vi "WaveformComponent, Append Pulse Center.vi"(0 "waveform in":waveform(dbl)={"t0"=timestamp(3474820848.0780005 s since 1904-01-01), "dt"=nan, "Y"=[]}, 1 "append parameters":T1={"offset"=0.5, "amplitude"=-2.0, "delay"=0.00019999999999999998, "leading edge"=0.0005, "pulse width"=0.0006, "trailing edge"=0.0005, "ref level %"=33.333} {"ref level %" format="%.3f"; "offset" format="%.3f"; "pulse width" format="%.1f"; "trailing edge" format="%.1f"; "amplitude" format="%.3f"; "delay" format="%.1f"; "leading edge" format="%.1f"}) -> (3 "waveform out":waveform(dbl)={"t0"=timestamp(-9593225999.921999 s since 1904-01-01), "dt"=nan, "Y"=[]})   [LabVIEW 2010]
uses:
  Pulse Parameters.ctl
panel:
  out "edge rate adjustment":dbl[unit] format="%.3p"
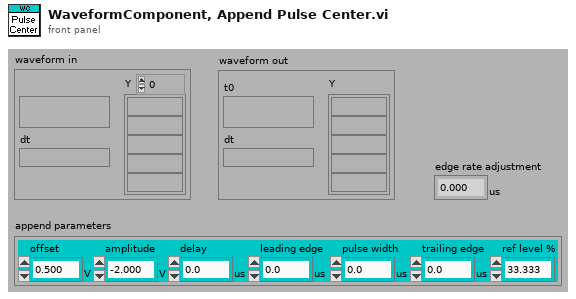
[diagram p1: front panel]
types:
  T1 = typedef "Pulse Parameters.ctl" = cluster{"offset":dbl[unit], "amplitude":dbl[unit], "delay":dbl[unit], "leading edge":dbl[unit], "pulse width":dbl[unit], "trailing edge":dbl[unit], "ref level %":dbl}
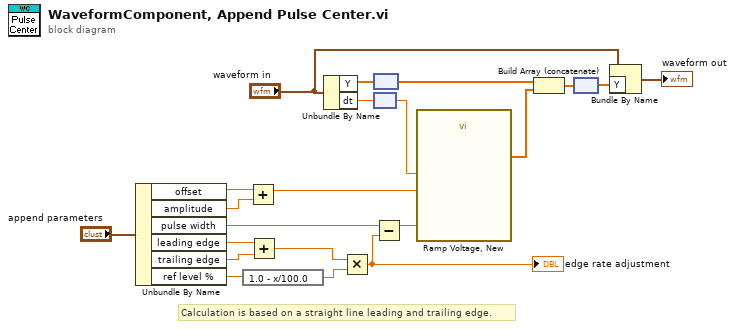
[diagram p0: block diagram]
diagram:
  # "Calculation is based on a straight line leading and trailing edge."
  n1 = Unbundle By Name("append parameters") -> ("offset"=w11:dbl[unit], "amplitude"=w12:dbl[unit], "pulse width"=w6:dbl[unit], "leading edge"=w2:dbl[unit], "trailing edge"=w3:dbl[unit], "ref level %"=w4:dbl)
  n2 = expression code="1.0 - x/100.0"(w4) -> (w9:dbl)
  n3 = Add(x=w11, y=w12) -> (x+y=w13:dbl[unit])
  n4 = Add(x=w2, y=w3) -> (x+y=w7:dbl[unit])
  n5 = Unbundle By Name("waveform in") -> ("Y"=w19:dbl[], "dt"=w17:dbl)
  n6 = Multiply(x=w7, y=w9) -> (x*y=w1:dbl[unit])
  "edge rate adjustment" <- w1
  n7 = node(w19) -> (w16:dbl[unit][])
  n8 = node(w17) -> (w8:dbl[unit])
  n9 = Subtract(x=w6, y=w1) -> (x-y=w5:dbl[unit])
  n10 = call "Ramp Voltage, New.vi"("offset (0.0)"=w13, "dt"=w8, "total time"=w5) -> ("ramp"=w20:dbl[unit][])  [unwired: 2 in]
  n11 = Build Array (concatenate)(w16, w20) -> (w15:dbl[unit][])
  n12 = node(w15) -> (w21:dbl[])
  n13 = Bundle By Name(cluster="waveform in", "Y"=w21) -> (→"waveform out":waveform(dbl))
